vi "POP_Set Font Size.vi"(8 "error in (no error)":errorcluster, 9 "Font Size":u32, 10 "TontName":string="Tahoma", 11 "Popup Cluster Ref":refnum<vi>) -> (0 "error out":errorcluster, 3 "dup ref out":refnum<vi>)   [LabVIEW 2016]
uses:
  Ctrls/POP_Data Type.ctl
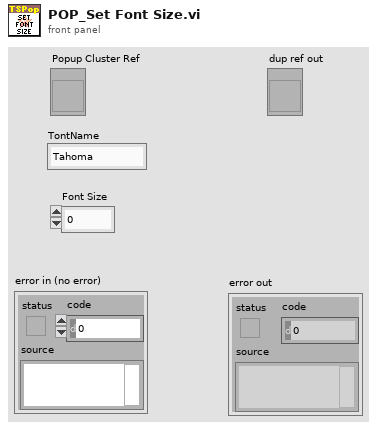
[diagram p1: front panel]
types:
  T1 = typedef "POP_Data Type.ctl" = enum16{"NO POPUP", "Unkown", "String", "Integer", "Float", "Color", "Boolean", "Ring", "Captioned String", "Captioned Integer", "Button Color", "2 Int Cluster", "4 Int Cluster", "6-Dbl Cluster", "Path", "Combox", "Time", "ShotCut String"}
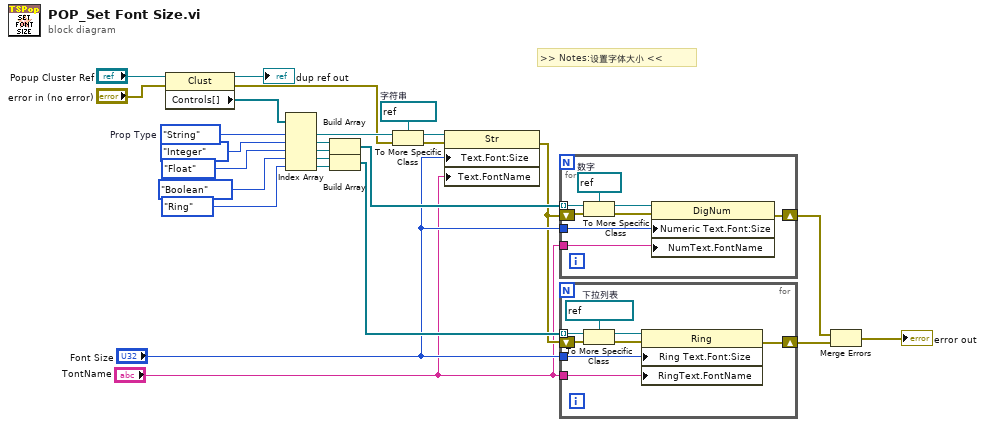
[diagram p0: block diagram]
diagram:
  w24 = refnum<vi> refnum  # 字符串
  w26 = POP_Data_Type."String"  # Prop Type
  # ">> Notes:设置字体大小 <<"
  n1 = property class="Clust"(reference="Popup Cluster Ref", error in="error in (no error)") -> (reference out=→"dup ref out":refnum<vi>, error out=w7:errorcluster, "Controls[]"=w10:refnum<vi>[])
  n2 = Index Array(array=w10, index #1=w26, index #2=POP_Data_Type."Integer" ("Prop Type"), index #3=POP_Data_Type."Float" ("Prop Type"), index #4=POP_Data_Type."Boolean" ("Prop Type"), index #5=POP_Data_Type."Ring" ("Prop Type")) -> (element #1=w25:refnum<vi>, element #2=w20:refnum<vi>, element #3=w19:refnum<vi>, element #4=w15:refnum<vi>, element #5=w14:refnum<vi>)
  n3 = Build Array(w20, w19) -> (w18:refnum<vi>[])
  n4 = Build Array(w15, w14) -> (w13:refnum<vi>[])
  n5 = To More Specific Class(target class=w24, reference=w25, error in=w7) -> (specific class reference=w23:refnum<vi>, error out=w6:errorcluster)
  n6 = property class="Str"(reference=w23, error in=w6, "Text.Font:Size"="Font Size", "Text.FontName"="TontName") -> (error out=w5:errorcluster)  [unwired: 1 out]
  n7 = for {
    tunnel: w18 -> [w32] mode=indexing
    tunnel: "Font Size" -> [w31]
    shift-right: [w28] -> w4
    shift-left: w5 -> [w30]
    tunnel: "TontName" -> [w27]
    w33 = refnum<vi> refnum  # 数字
    n8 = To More Specific Class(target class=w33, reference=w32, error in=w30) -> (specific class reference=w34:refnum<vi>, error out=w29:errorcluster)
    n9 = property class="DigNum"(reference=w34, error in=w29, "Numeric Text.Font:Size"=w31, "NumText.FontName"=w27) -> (error out=w28:errorcluster)  [unwired: 1 out]
  }
  n10 = for {
    tunnel: w13 -> [w40] mode=indexing
    tunnel: "Font Size" -> [w39]
    shift-right: [w36] -> w3
    shift-left: w5 -> [w38]
    tunnel: "TontName" -> [w35]
    w41 = refnum<vi> refnum  # 下拉列表
    n11 = To More Specific Class(target class=w41, reference=w40, error in=w38) -> (specific class reference=w42:refnum<vi>, error out=w37:errorcluster)
    n12 = property class="Ring"(reference=w42, error in=w37, "Ring Text.Font:Size"=w39, "RingText.FontName"=w35) -> (error out=w36:errorcluster)  [unwired: 1 out]
  }
  n13 = Merge Errors(w4, w3) -> (→"error out":errorcluster)
